vi "Check Threads For Errors.vi"(8 "error in (no error)":errorcluster, 11 "Framework in":refnum<class "Framework.lvclass">) -> (0 "error out":errorcluster, 1 "private thread error":bool, 2 "public thread error":bool, 3 "Framework out":refnum<class "Framework.lvclass">)   [LabVIEW 2020, in "DSF Core.lvlib" / "Framework.lvclass"]
uses:
  Framework.lvclass
  Thread/Thread State.ctl
  Thread/Thread.lvclass
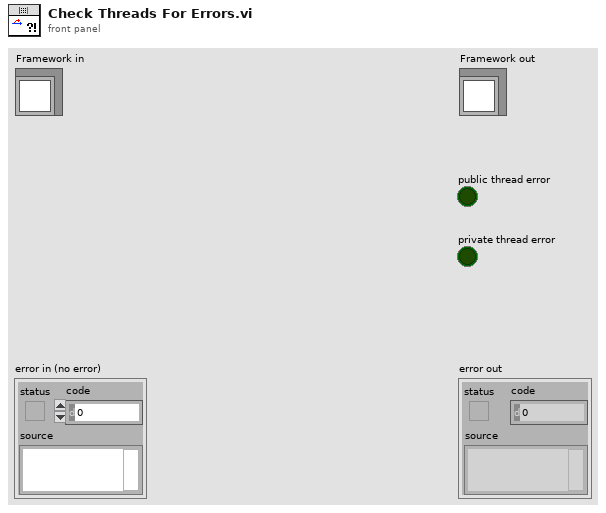
[diagram p1: front panel]
types:
  T1 = typedef "DSF Core.lvlib/Thread.lvclass/Thread State.ctl" = enum8{"Idle", "Running", "Error", "Shut Down"}
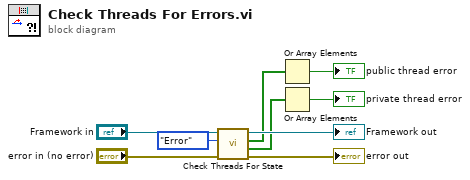
[diagram p0: block diagram]
diagram:
  n1 = call "Check Threads For State.vi"("error in (no error)"="error in (no error)", "state"=Thread_State."Error" ("check for state"), "Framework in"="Framework in") -> ("error out"=→"error out":errorcluster, "private threads equal"=w3:bool[], "public threads equal"=w4:bool[], "Framework out"=→"Framework out":refnum<class "Framework.lvclass">)  [unwired: 5 in]
  n2 = Or Array Elements(Boolean array=w4) -> (logical OR=→"public thread error":bool)
  n3 = Or Array Elements(Boolean array=w3) -> (logical OR=→"private thread error":bool)
